vi "arraySwitching.vi"() -> ()   [LabVIEW 2018]
panel:
  out "Array 2":i32[](array[numeric])
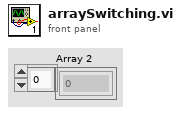
[diagram p1: front panel]
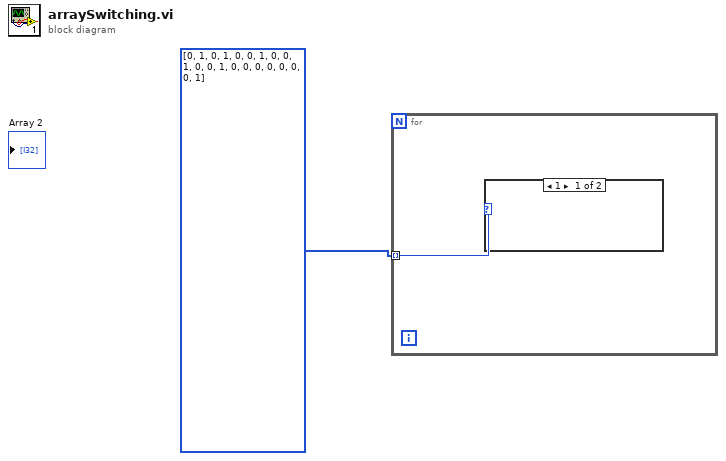
[diagram p0: block diagram]
diagram:
  n1 = for {
    tunnel: i32[] [0, 1, 0, 1, 0, 0, 1, 0, 0, 1, 0, 0, 1, 0, 0, 0, 0, 0, 0, 0, 1] -> [w2] mode=indexing
    n2 = case shown="1" w2 {
      frame 1 {
      }
      frame 0 {
      }
    }
  }
